vi "Set View Reference.vi"(8 "error in (no error)":errorcluster, 9 "VI Reference":refnum<vi>, 10 "View Name":string, 11 "UI Controller in":refnum<class "UI Controller.lvclass">) -> (0 "error out":errorcluster, 3 "UI Controller out":refnum<class "UI Controller.lvclass">)   [LabVIEW 2020, in "UI Controller.lvlib" / "UI Controller.lvclass"]
uses:
  UI Controller.lvclass
  C:/Program Files/National Instruments/LabVIEW 2020/vi.lib/ActorFrameworkMVC/Abstract Controller/Abstract Controller/Abstract Controller.lvclass
  <vilib>/ActorFrameworkMVC/View Controller/View Controller/View Controller.lvclass
  <vilib>/ActorFrameworkMVC/Abstract Controller/Abstract Controller/Abstract Controller.lvclass
panel:
  # "NOTICE -- YOU MUST LEAVE THIS NOTICE IN PLACE.\n\nCopyright (c) 2017, LIANG LIU Shawn.Liu.cn@gmail.com\nAll rights reserved.\n\nRedistribution and use in source and binary forms, with or without modification, are permitted provided that the following conditions are met:\n-Redistributions of source code must retain the above copyright notice, this list of conditions and the following disclaimer.\n-Redistributions in binary form must reproduce the above copyright notice, this list of conditions and the following disclaimer in the documentation and/or other materials provided with the distribution.\n-Neither the name of the eLp nor the names of its contributors may be used to endorse or promote products derived from this software without specific prior written permission.\n\nTHIS SOFTWARE IS PROVIDED BY THE COPYRIGHT HOLDERS AND CONTRIBUTORS \"AS IS\" AND ANY EXPRESS OR IMPLIED WARRANTIES, INCLUDING, BUT NOT LIMITED TO, THE IMPLIED WARRANTIES OF MERCHANTABILITY AND FITNESS FOR A PARTICULAR PURPOSE ARE DISCLAIMED. IN NO EVENT SHALL THE COPYRIGHT HOLDER OR CONTRIBUTORS BE LIABLE FOR ANY DIRECT, INDIRECT, INCIDENTAL, SPECIAL, EXEMPLARY, OR CONSEQUENTIAL DAMAGES (INCLUDING, BUT NOT LIMITED TO, PROCUREMENT OF SUBSTITUTE GOODS OR SERVICES; LOSS OF USE, DATA, OR PROFITS; OR BUSINESS INTERRUPTION) HOWEVER CAUSED AND ON ANY THEORY OF LIABILITY, WHETHER IN CONTRACT, STRICT LIABILITY, OR TORT (INCLUDING NEGLIGENCE OR OTHERWISE) ARISING IN ANY WAY OUT OF THE USE OF THIS SOFTWARE, EVEN IF ADVISED OF THE POSSIBILITY OF SUCH DAMAGE."
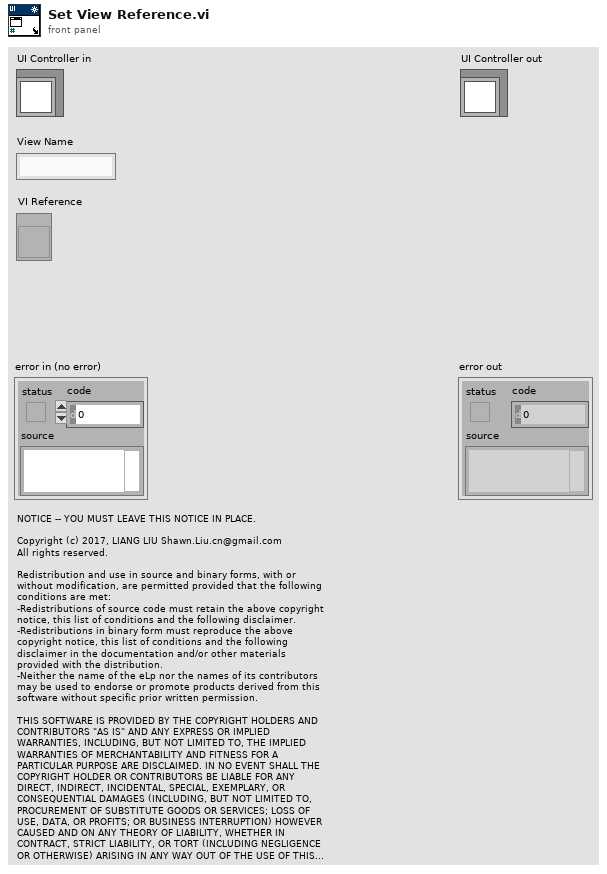
[diagram p1: front panel]
types:
  T1 = typedef "LVRectTypeDef.ctl" = cluster{"Left":i16, "Top":i16, "Right":i16, "Bottom":i16}
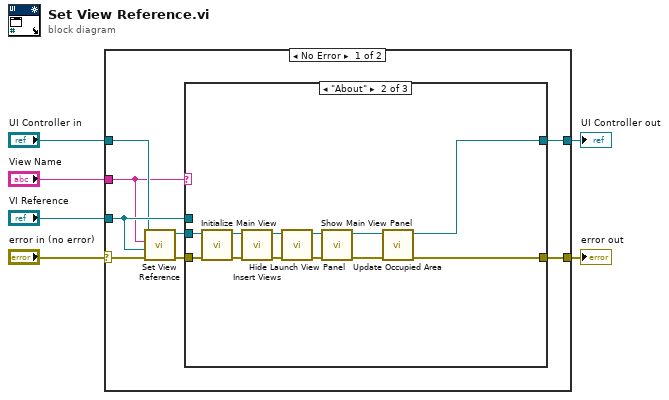
[diagram p0: block diagram]
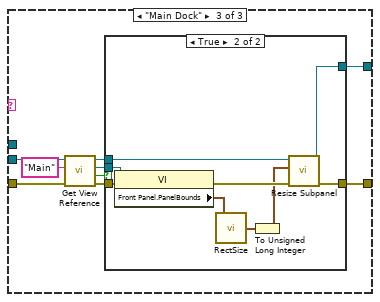
[diagram p3: hidden frame]
diagram:
  n1 = case shown="No Error" "error in (no error)" {
    selector: "error in (no error)" -> [w14 w50]
    tunnel: "VI Reference" -> [w13 _]
    tunnel: "UI Controller in" -> [w12 w49]
    tunnel: "View Name" -> [w11 _]
    tunnel: [w10 w50] -> w2
    tunnel: [w9 w49] -> w1
    frame No Error {
      n2 = call-parent "Set View Reference.vi"("error in (no error)"=w14, "VI Reference"=w13, "View Name"=w11, "Abstract Controller in"=w12) -> ("error out"=w8:errorcluster, "Abstract Controller out"=w7:refnum<class "UI Controller.lvclass">)  [unwired: 6 in]
      n3 = case shown="\"About\"" w11 {
        tunnel: w8 -> [w16 w28 w37]
        tunnel: w7 -> [w15 w25 w33]
        tunnel: [w16 w19 w36] -> w10
        tunnel: [w15 w17 w35] -> w9
        tunnel: w13 -> [_ _ _]
        frame Default {
        }
        frame "About" {
          n4 = call "Initialize Main View.vi"("error in (no error)"=w28, "UI Controller in"=w25) -> ("error out"=w26:errorcluster, "UI Controller out"=w24:refnum<class "UI Controller.lvclass">)  [unwired: 8 in]
          n5 = call "Insert Views.vi"("error in (no error)"=w26, "UI Controller in"=w24) -> ("error out"=w27:errorcluster, "UI Controller out"=w20:refnum<class "UI Controller.lvclass">)  [unwired: 8 in]
          n6 = call "Hide Launch View Panel.vi"("error in (no error)"=w27, "UI Controller in"=w20) -> ("error out"=w23:errorcluster, "UI Controller out"=w21:refnum<class "UI Controller.lvclass">)  [unwired: 8 in]
          n7 = call "Show Main View Panel.vi"("error in (no error)"=w23, "UI Controller in"=w21) -> ("error out"=w22:errorcluster, "UI Controller out"=w18:refnum<class "UI Controller.lvclass">)  [unwired: 8 in]
          n8 = call "Update Occupied Area.vi"("error in (no error)"=w22, "UI Controller in"=w18) -> ("error out"=w19:errorcluster, "UI Controller out"=w17:refnum<class "UI Controller.lvclass">)  [unwired: 8 in]
        }
        frame "Main Dock" {
          n9 = call <vilib>:"Get View Reference.vi"("error in (no error)"=w37, "View Name"="Main", "Abstract Controller in"=w33) -> ("error out"=w34:errorcluster, "Found?"=w29:bool, "VI Reference"=w31:refnum<vi>, "Abstract Controller out"=w32:refnum<class "UI Controller.lvclass">)  [unwired: 5 in]
          n10 = case shown="True" w29 {
            tunnel: [w38 w47] -> w36
            tunnel: [w39 w45] -> w35
            tunnel: w34 -> [w38 w42]
            tunnel: w32 -> [w39 w41]
            tunnel: w31 -> [_ w40]
            frame False {
            }
            frame True {
              n11 = property class="VI"(reference=w40, error in=w42) -> (error out=w48:errorcluster, "Front Panel.PanelBounds"=w44:T1)  [unwired: 1 out]
              n12 = call <vilib>:"RectSize.vi"("rect"=w44) -> ("point"=w46:cluster{"x":i16, "y":i16})
              n13 = To Unsigned Long Integer(number=w46) -> (unsigned 32bit integer=w43:cluster{"x":u32, "y":u32})
              n14 = call "Resize Subpanel.vi"("error in (no error)"=w48, "Subpanel Size"=w43, "UI Controller in"=w41) -> ("error out"=w47:errorcluster, "UI Controller out"=w45:refnum<class "UI Controller.lvclass">)  [unwired: 7 in]
            }
          }
        }
      }
    }
    frame Error {
    }
  }
  "error out" <- w2
  "UI Controller out" <- w1
